vi "Norm Coords to Voltage.vi"(10 "AOD Configuration":T1={"Physical Channel"="Dev1/ao0:1", "Maximum Value"=10.0, "Minimum Value"=1.0, "Update Rate"=192000.0} {"Update Rate" format="%0.2f"; "Minimum Value" format="%0.2f"; "Maximum Value" format="%0.2f"}, 11 "coords in":dbl[](array[numeric])) -> (3 "voltage out":dbl[](array[numeric]))   [LabVIEW 2015, in "AOD.lvlib"]
uses:
  AOD.lvlib
  AOD Configuration.ctl
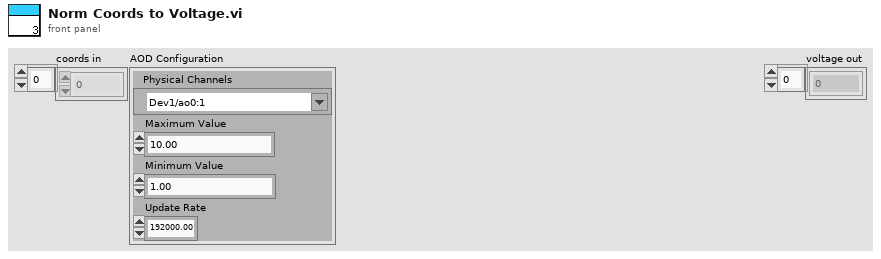
[diagram p1: front panel]
types:
  T1 = typedef "AOD.lvlib/AOD Configuration.ctl" = cluster{"Physical Channel":tag, "Maximum Value":dbl, "Minimum Value":dbl, "Update Rate":dbl}
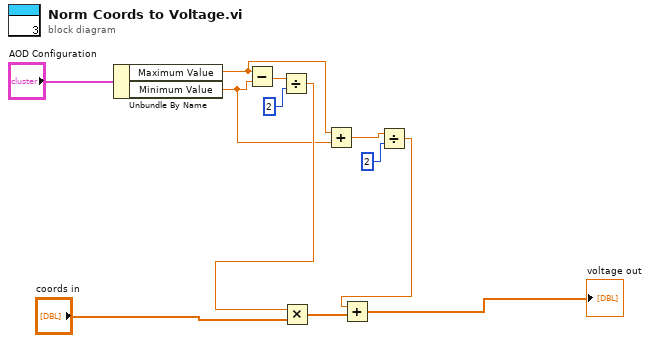
[diagram p0: block diagram]
diagram:
  n1 = Unbundle By Name("AOD Configuration") -> ("Maximum Value"=w5:dbl, "Minimum Value"=w4:dbl)
  n2 = Subtract(x=w5, y=w4) -> (x-y=w8:dbl)
  n3 = Divide(x=w8, y=2) -> (x/y=w6:dbl)
  n4 = Multiply(x=w6, y="coords in") -> (x*y=w12:dbl[])
  n5 = Add(x=w5, y=w4) -> (x+y=w3:dbl)
  n6 = Divide(x=w3, y=2) -> (x/y=w1:dbl)
  n7 = Add(x=w1, y=w12) -> (x+y=→"voltage out":dbl[])
